vi "update_sample_list.vi"(11 "SampleList Ref":refnum<vi>) -> ()   [LabVIEW 2020]
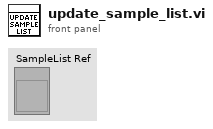
[diagram p1: front panel]
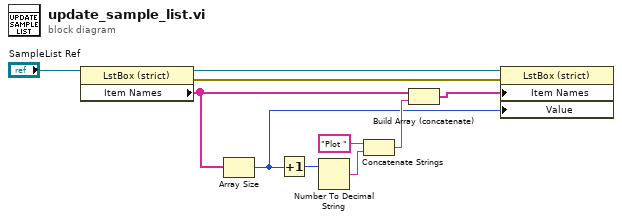
[diagram p0: block diagram]
diagram:
  n1 = property class="LstBox (strict)"(reference="SampleList Ref") -> (reference out=w8:refnum<vi>, error out=w9:errorcluster, "Item Names"=w5:string[])  [unwired: 1 in]
  n2 = Array Size(array=w5) -> (size(s)=w1:i32)
  n3 = Increment(x=w1) -> (x+1=w2:i32)
  n4 = Number To Decimal String(number=w2) -> (decimal integer string=w6:string)  [unwired: 1 in]
  n5 = Concatenate Strings("Plot ", w6) -> (w4:string)
  n6 = Build Array (concatenate)(w5, w4) -> (w3:string[])
  n7 = property class="LstBox (strict)"(reference=w8, error in=w9, "Item Names"=w3, "Value"=w1) -> ()  [unwired: 2 out]
